vi "未命名 1.vi"() -> ()   [LabVIEW 2019]
uses:
  <vilib>/Instr/_visa.llb/VISA Configure Serial Port (Instr).vi
panel:
  out "输出簇":T1
  out "校验位":i32
  out "停止位":i32
  out "数据位":i32
  out "波特率":i32
  out "VISA资源名称":refnum<visa-resource-name>
  out "VISA resource name out":refnum<visa-resource-name>
  in  "串口配置":T2={"VISA资源名称"="COM1", "波特率"=9600, "数据位"=8, "校验"=enum."None", "停止位"=enum."2.0"} {"数据位" min=5 max=8 step=1; "波特率" items=["75"=75, "110"=110, "134"=134, "150"=150, "300"=300, "600"=600, "1200"=1200, "1800"=1800, "2400"=2400, "4800"=4800, "7200"=7200, "9600"=9600, "14400"=14400, "19200"=19200, "28800"=28800, "38400"=38400, "56000"=56000, "57600"=57600, "115200"=115200, "128000"=128000, "230400"=230400]}
  in  "停止":bool
  # "串口号："
  # "停止位："
  # "校验位"
  # "数据位："
  # "波特率："
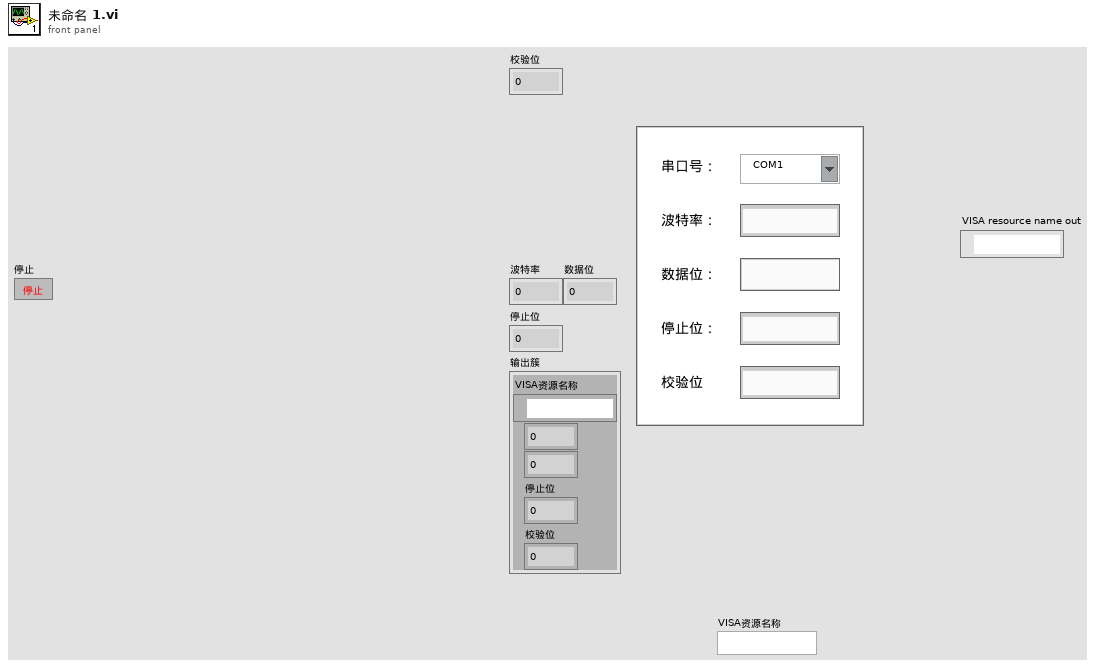
[diagram p1: front panel]
types:
  T1 = cluster{"VISA资源名称":refnum<visa-resource-name>, i32, i32, "停止位":i32, "校验位":i32}
  T2 = cluster{"VISA资源名称":refnum<visa-resource-name>, "波特率":u32, "数据位":u16, "校验":enum16{"None", "Odd", "Even", "Mark", "Space"}, "停止位":enum16{"1.0", "1.5", "2.0"}}
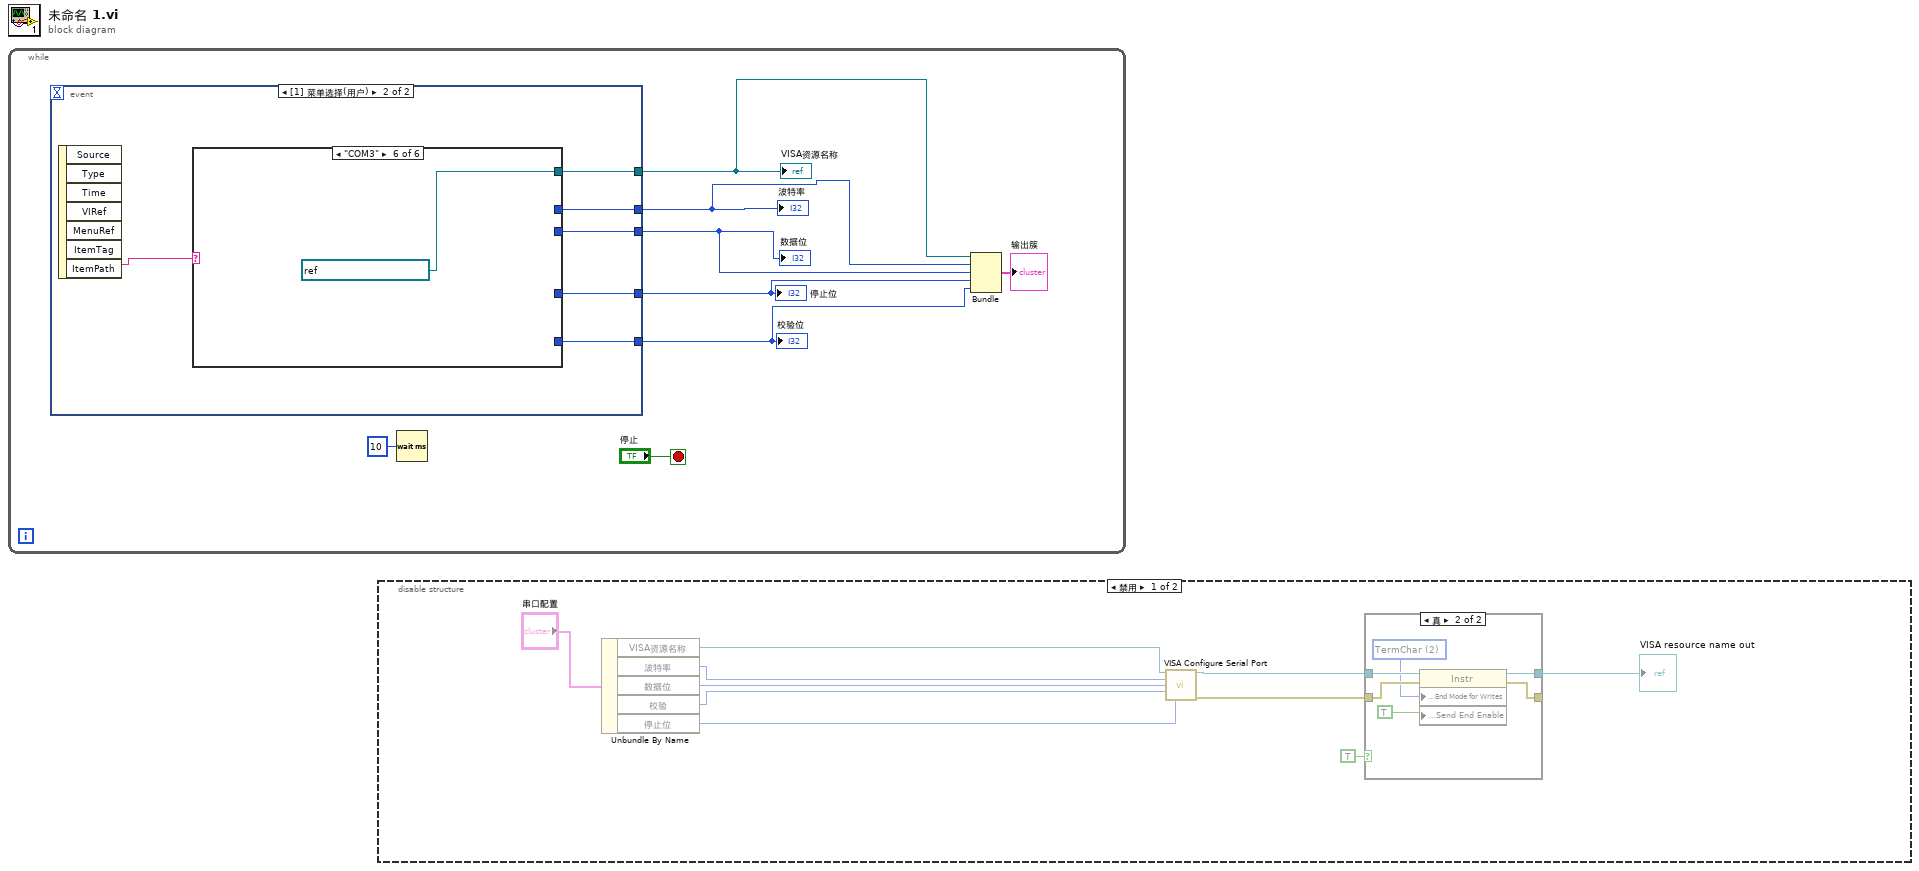
[diagram p0: block diagram]
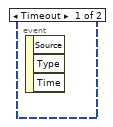
[diagram p4: hidden frame]
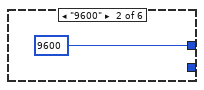
[diagram p6: hidden frame]
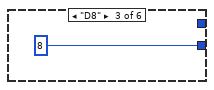
[diagram p7: hidden frame]
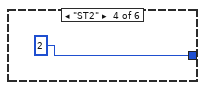
[diagram p8: hidden frame]
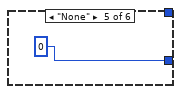
[diagram p9: hidden frame]
diagram:
  n1 = while {
    stop <- "停止" stop-if-true
    n2 = event shown="[1] 菜单选择(用户)" {
      selector: _ -> [_ _]
      dyn-events: _ -> [_ _]
      timeout: _ -> [_ _]
      tunnel: [_ w13] -> w6
      tunnel: [_ w12] -> w5
      tunnel: [_ w11] -> w4
      tunnel: [_ w10] -> w3
      tunnel: [_ w9] -> w2
      event Timeout {
        n3 = event-data() -> ()  [unwired: 1 in, 3 out]
      }
      event Menu Selection (User) {
        n4 = event-data() -> ("ItemTag"=w14:string)  [unwired: 1 in, 6 out]
        n5 = case shown="\"COM3\"" w14 {
          tunnel: [_ _ _ _ _ refnum<visa-resource-name> "COM3" ("VISA资源名称")] -> w13
          tunnel: [_ 9600 _ _ _ _] -> w12
          tunnel: [_ _ 8 _ _ _] -> w11
          tunnel: [_ _ _ 2 ("停止位") _ _] -> w10
          tunnel: [_ _ _ _ 0 ("校验位") _] -> w9
          frame "假", Default {
          }
          frame "9600" {
          }
          frame "D8" {
          }
          frame "ST2" {
          }
          frame "None" {
          }
          frame "COM3" {
          }
        }
      }
    }
    "VISA资源名称" <- w6
    "波特率" <- w5
    "数据位" <- w4
    "停止位" <- w3
    "校验位" <- w2
    n6 = Wait (ms)(milliseconds to wait=u32 10 ("等待时间（毫秒）")) -> ()  [unwired: 1 out]
    n7 = Bundle("VISA资源名称"=w6, w5, w4, "停止位"=w3, "校验位"=w2) -> (→"输出簇":T1)  [unwired: 1 in]
  }
  n8 = disable-structure shown="禁用" {
    frame Disabled {
      n9 = Unbundle By Name("串口配置") -> ("VISA资源名称"=w21:refnum<visa-resource-name>, "波特率"=w28:u32, "数据位"=w27:u16, "校验"=w26:enum16{"None", "Odd", "Even", "Mark", "Space"}, "停止位"=w20:enum16{"1.0", "1.5", "2.0"})
      n10 = call-poly "VISA Configure Serial Port"("VISA resource name"=w21, "baud rate (9600)"=w28, "data bits (8)"=w27, "parity (0:none)"=w26, "stop bits (10: 1 bit)"=w20) -> ("VISA resource name out"=w24:refnum<visa-resource-name>, "error out"=w23:errorcluster)  [unwired: 5 in, 4 out]
      n11 = case shown="真" TRUE {
        tunnel: w24 -> [w30 w37]
        tunnel: w23 -> [w31 w36]
        tunnel: [w30 w35] -> w25
        tunnel: [w31 w34] -> _
        frame False {
        }
        frame True {
          w33 = u16 2 items=["None", "LastBit", "TermChar", "Break"] ("Serial Settings:Serial End Mode for Writes")
          n12 = property class="Instr"(reference=w37, error in=w36, "Serial Settings:End Mode for Writes"=w33, "Message Based Settings:Send End Enable"=TRUE) -> (reference out=w35:refnum<visa-resource-name>, error out=w34:errorcluster)
        }
      }
      "VISA resource name out" <- w25
    }
    frame Enabled {
    }
  }
